vi "MakeThetaLabels.vi"(1 "ticsAndGrids":T1={"tics"={"ticMin"=0.0, "ticStep"=0.0, "ticMax"=0.0, "minorDivsPerMajor"=2, "ticSpacing"=enum."Auto Tics", "ticPosition"=enum."Inside, no mirror"}, "Grids"={"Gridlines"=enum."Major grid", "Zeroaxis"=enum."No zero axis"}, "Mapping"=enum."Lin"}) -> (0 "Theta Label Command String":string[](array[string]))   [LabVIEW 2022 SP3]
uses:
  ticsAndGrids.ctl
  tics.ctl
  grids.ctl
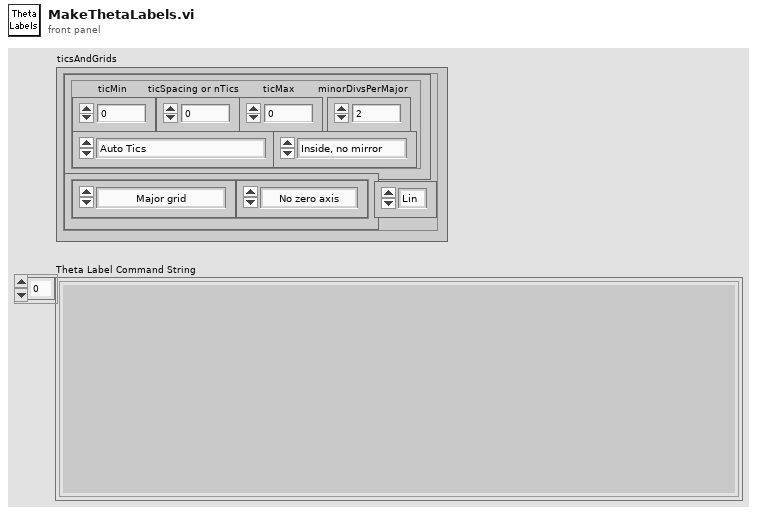
[diagram p1: front panel]
types:
  T1 = typedef "ticsAndGrids.ctl" = cluster{"tics":T2, "Grids":T3, "Mapping":enum8{"Lin", "Log"}}
  T2 = typedef "tics.ctl" = cluster{"ticMin":dbl, "ticStep":dbl, "ticMax":dbl, "minorDivsPerMajor":i32, "ticSpacing":enum16{"Auto Tics", "Fixed spacing", "Fixed Minimum and Spacing", "Start, Spacing and Maximum", "Approx n Tics (rounded)"}, "ticPosition":enum16{"Inside, no mirror", "Inside, mirrored", "Outside, no mirror", "Outside, mirrored", "Invisible"}}
  T3 = typedef "grids.ctl" = cluster{"Gridlines":enum16{"No grids", "Major grid", "Minor grid", "Major and Minor"}, "Zeroaxis":enum16{"No zero axis", "Show zero axis"}}
  T4 = enum16{"Auto Tics", "Fixed spacing", "Fixed Minimum and Spacing", "Start, Spacing and Maximum", "Approx n Tics (rounded)"}
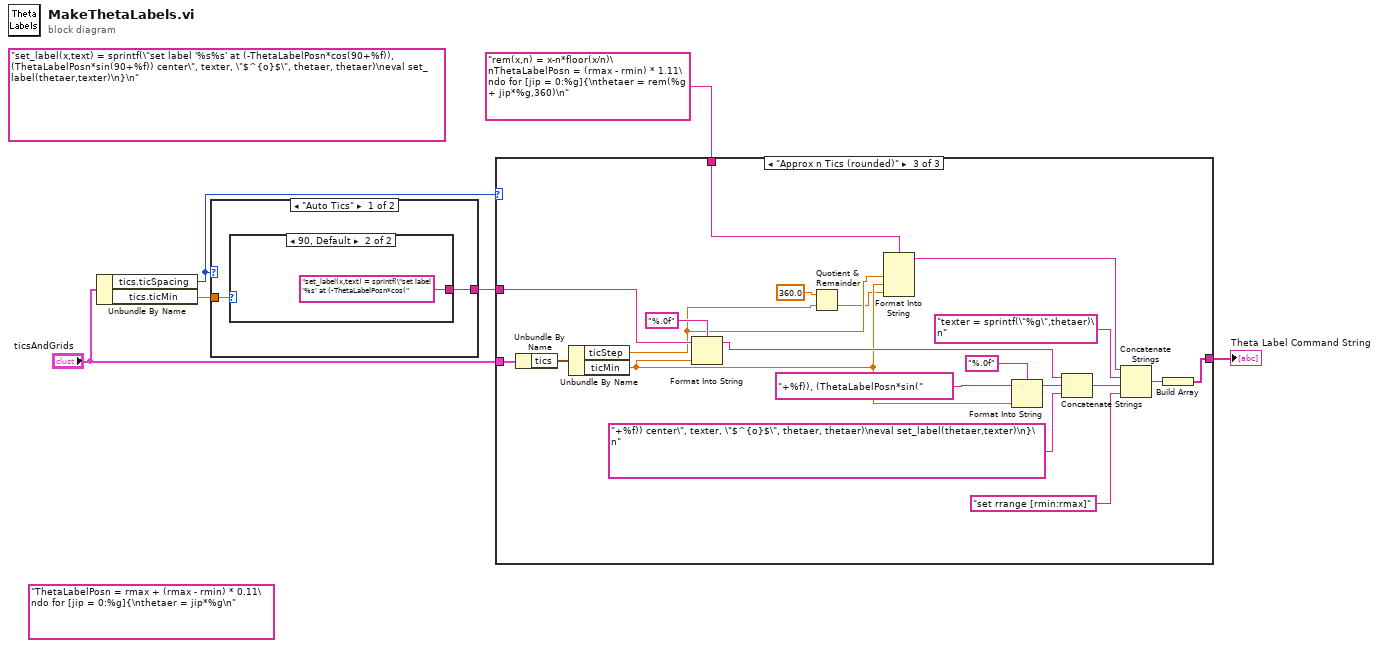
[diagram p0: block diagram]
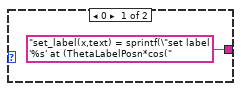
[diagram p2: hidden frame]
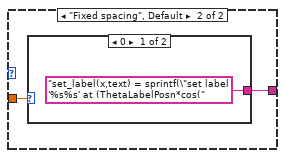
[diagram p3: hidden frame]
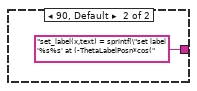
[diagram p4: hidden frame]
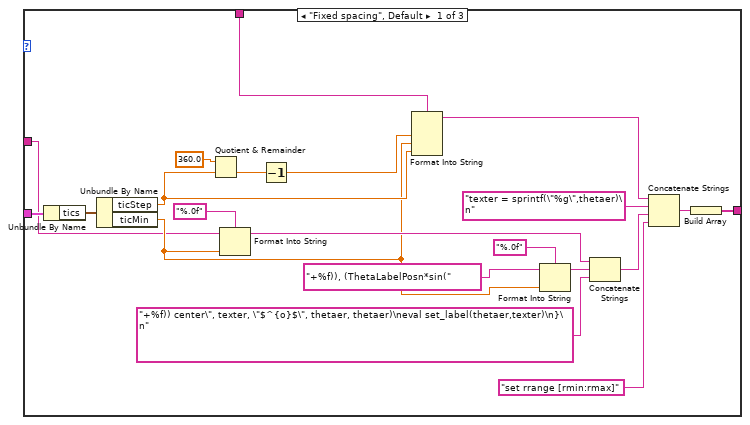
[diagram p5: hidden frame]
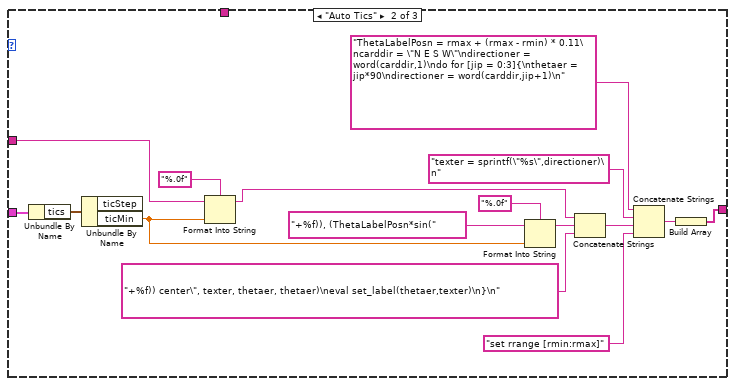
[diagram p6: hidden frame]
diagram:
  (unwired) "ThetaLabelPosn = rmax + (rmax - rmin) * 0.11\ndo for [jip = 0:%g]{\nthetaer = jip*%g\n"
  (unwired) "set_label(x,text) = sprintf(\"set label '%s%s' at (-ThetaLabelPosn*cos(90+%f)), (ThetaLabelPosn*sin(90+%f)) center\", texter, \"$^{o}$\", thetaer, thetaer)\neval set_label(thetaer,texter)\n}\n"
  n1 = Unbundle By Name("ticsAndGrids") -> ("tics.ticSpacing"=w2:T4, "tics.ticMin"=w4:dbl)
  n2 = case shown="\"Auto Tics\"" w2 {
    tunnel: w4 -> [w8 w12]
    tunnel: [w7 w11] -> w3
    frame "Auto Tics" {
      n3 = case shown="90, Default" w8 {
        tunnel: ["set_label(x,text) = sprintf(\"set label '%s' at (ThetaLabelPosn*cos(" "set_label(x,text) = sprintf(\"set label '%s' at (-ThetaLabelPosn*cos("] -> w7
        frame 0 {
        }
        frame 90, Default {
        }
      }
    }
    frame "Fixed spacing", Default {
      n4 = case shown="0" w12 {
        tunnel: ["set_label(x,text) = sprintf(\"set label '%s%s' at (ThetaLabelPosn*cos(" "set_label(x,text) = sprintf(\"set label '%s%s' at (-ThetaLabelPosn*cos("] -> w11
        frame 0 {
        }
        frame 90, Default {
        }
      }
    }
  }
  n5 = case shown="\"Approx n Tics (rounded)\"" w2 {
    tunnel: "ticsAndGrids" -> [w19 w39 w59]
    tunnel: [w18 w38 w58] -> w5
    tunnel: w3 -> [w16 w36 w56]
    tunnel: "rem(x,n) = x-n*floor(x/n)\nThetaLabelPosn = (rmax - rmin) * 1.11\ndo for [jip = 0:%g]{\nthetaer = rem(%g + jip*%g,360)\n" -> [w15 _ w52]
    frame "Fixed spacing", Default {
      n6 = Unbundle By Name(w19) -> ("tics"=w29:T2)
      n7 = Unbundle By Name(w29) -> ("ticStep"=w33:dbl, "ticMin"=w17:dbl)
      n8 = Quotient & Remainder(x=360.0, y=w33) -> (floor(x/y)=w31:dbl)  [unwired: 1 out]
      n9 = Format Into String(format string="%.0f", initial string=w16, w17) -> (resulting string=w23:string)  [unwired: 1 in, 1 out]
      n10 = Decrement(x=w31) -> (x-1=w32:dbl)
      n11 = Format Into String(format string=w15, w32, w17, w33) -> (resulting string=w34:string)  [unwired: 2 in, 1 out]
      n12 = Format Into String(format string="%.0f", initial string="+%f)), (ThetaLabelPosn*sin(", w17) -> (resulting string=w22:string)  [unwired: 1 in, 1 out]
      n13 = Concatenate Strings(w23, w22, "+%f)) center\", texter, \"$^{o}$\", thetaer, thetaer)\neval set_label(thetaer,texter)\n}\n") -> (w20:string)
      n14 = Concatenate Strings(w34, "texter = sprintf(\"%g\",thetaer)\n" ("string"), w20, "set rrange [rmin:rmax]" ("string")) -> (w28:string)
      n15 = Build Array(w28) -> (w18:string[])
    }
    frame "Auto Tics" {
      n16 = Unbundle By Name(w39) -> ("tics"=w50:T2)
      n17 = Unbundle By Name(w50) -> ("ticMin"=w40:dbl)  [unwired: 1 out]
      n18 = Format Into String(format string="%.0f", initial string=w36, w40) -> (resulting string=w44:string)  [unwired: 1 in, 1 out]
      n19 = Format Into String(format string="%.0f", initial string="+%f)), (ThetaLabelPosn*sin(", w40) -> (resulting string=w43:string)  [unwired: 1 in, 1 out]
      n20 = Concatenate Strings(w44, w43, "+%f)) center\", texter, thetaer, thetaer)\neval set_label(thetaer,texter)\n}\n") -> (w41:string)
      n21 = Concatenate Strings("ThetaLabelPosn = rmax + (rmax - rmin) * 0.11\ncarddir = \"N E S W\"\ndirectioner = word(carddir,1)\ndo for [jip = 0:3]{\nthetaer = jip*90\ndirectioner = word(carddir,jip+1)\n", "texter = sprintf(\"%s\",directioner)\n" ("string"), w41, "set rrange [rmin:rmax]" ("string")) -> (w49:string)
      n22 = Build Array(w49) -> (w38:string[])
    }
    frame "Approx n Tics (rounded)" {
      n23 = Unbundle By Name(w59) -> ("tics"=w69:T2)
      n24 = Unbundle By Name(w69) -> ("ticStep"=w55:dbl, "ticMin"=w57:dbl)
      n25 = Format Into String(format string="%.0f", initial string=w56, w57) -> (resulting string=w63:string)  [unwired: 1 in, 1 out]
      n26 = Quotient & Remainder(x=360.0, y=w55) -> (floor(x/y)=w53:dbl)  [unwired: 1 out]
      n27 = Format Into String(format string=w52, w55, w57, w53) -> (resulting string=w70:string)  [unwired: 2 in, 1 out]
      n28 = Format Into String(format string="%.0f", initial string="+%f)), (ThetaLabelPosn*sin(", w57) -> (resulting string=w62:string)  [unwired: 1 in, 1 out]
      n29 = Concatenate Strings(w63, w62, "+%f)) center\", texter, \"$^{o}$\", thetaer, thetaer)\neval set_label(thetaer,texter)\n}\n") -> (w60:string)
      n30 = Concatenate Strings(w70, "texter = sprintf(\"%g\",thetaer)\n" ("string"), w60, "set rrange [rmin:rmax]" ("string")) -> (w68:string)
      n31 = Build Array(w68) -> (w58:string[])
    }
  }
  "Theta Label Command String" <- w5
